vi "Main.vi"(8 "error in":errorcluster caption="entrée d'erreur") -> (0 "error out":errorcluster caption="sortie d'erreur")   [LabVIEW 2026]
uses:
  FGV/TypeDef_Array_ChannelCluster.ctl
  FGV/TypeDef_FGV.ctl
panel:
  in  "Arrêter":bool
  in  "Channel_Cluster_Array IN":T1 {"Filter" items=["447/60", "475/35", "525/50", "600/37", "647/57", "647LP"]; "Exposure time (s)" min=0.0 max=5.0 step=0.01; "Power (%)" max=100 step=1}
  out "Waveform Graph":waveform(dbl)[](graph)=[{"t0"=timestamp(0 s since 1904-01-01), "dt"=1e-05, "Y"=array[75000 elements]}, {"t0"=timestamp(0 s since 1904-01-01), "dt"=1e-05, "Y"=array[75000 elements]}, {"t0"=timestamp(0 s since 1904-01-01), "dt"=1e-05, "Y"=array[75000 elements]}, {"t0"=timestamp(0 s since 1904-01-01), "dt"=1e-05, "Y"=array[75000 elements]}]
  out "DO WF OUT":digitalwaveform(graph)
  out "Waveform Graph 2":waveform(dbl)[](graph)=[{"t0"=timestamp(0 s since 1904-01-01), "dt"=1e-05, "Y"=array[75000 elements]}, {"t0"=timestamp(0 s since 1904-01-01), "dt"=1e-05, "Y"=array[75000 elements]}, {"t0"=timestamp(0 s since 1904-01-01), "dt"=1e-05, "Y"=array[75000 elements]}]
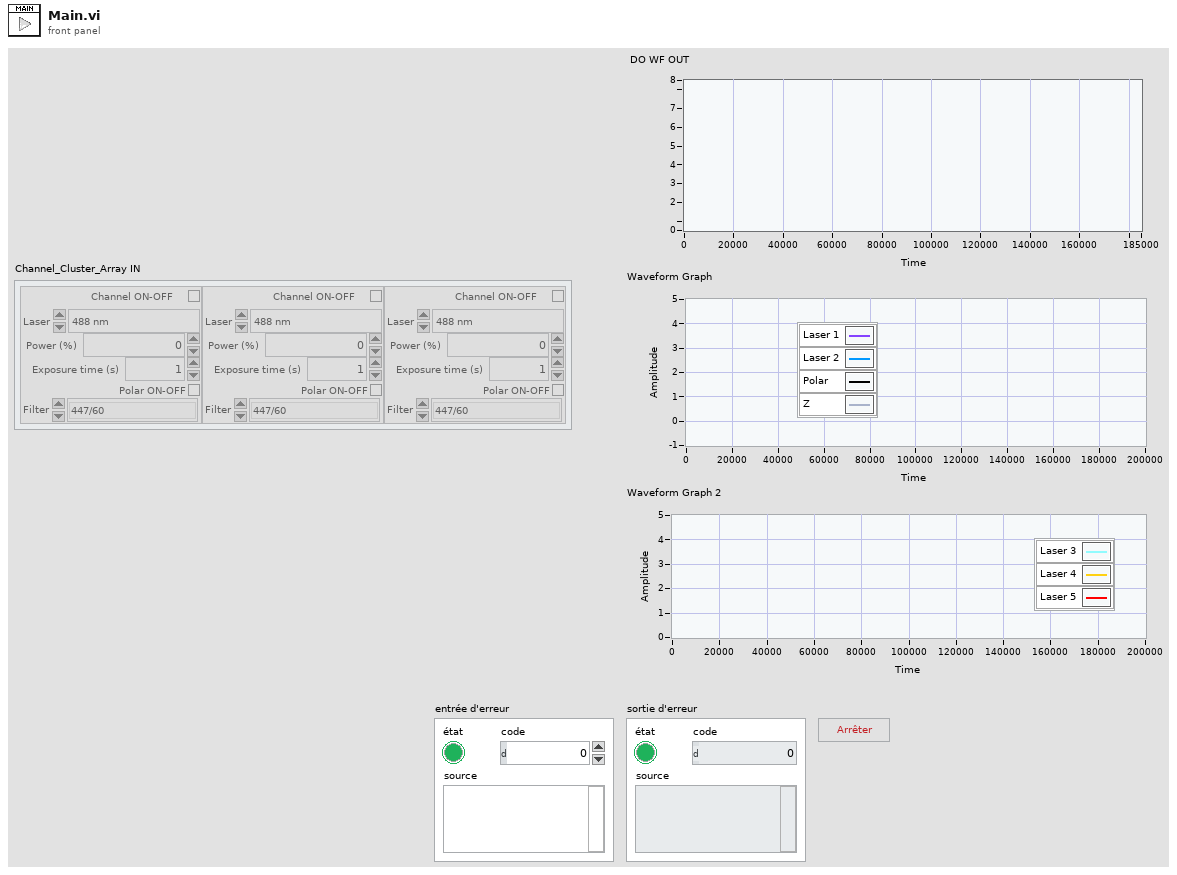
[diagram p1: front panel]
types:
  T1 = typedef "TypeDef_Array_ChannelCluster.ctl" = cluster{"Laser":enum16{"405 nm", "455 nm", "488 nm", "561 nm", "640 nm"}, "Power (%)":u8, "Exposure time (s)":dbl, "Channel ON-OFF":bool, "Polar ON-OFF":bool, "Filter":u16}[]
  T2 = typedef "TypeDef_FGV.ctl" = enum16{"Initialize", "Write", "Read", "Read_File", "Write_to_File"}
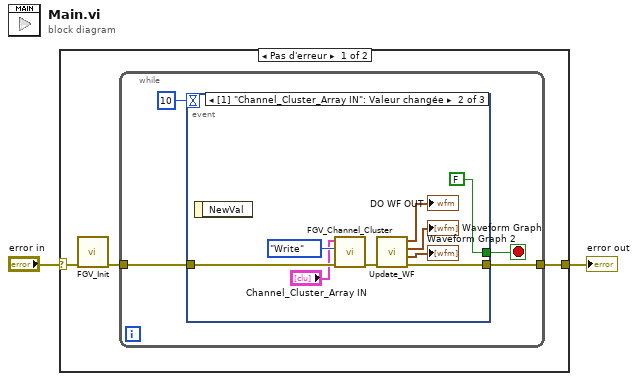
[diagram p0: block diagram]
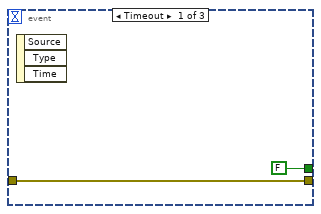
[diagram p2: hidden frame]
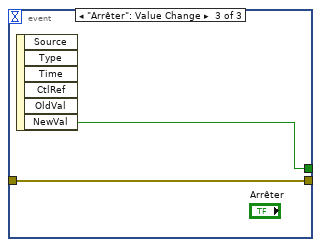
[diagram p3: hidden frame]
diagram:
  n1 = case shown="Pas d'erreur" "error in" {
    selector: "error in" -> [w3 w23]
    tunnel: [w5 w23] -> w1
    frame No Error {
      n2 = call "FGV_Init.vi"("error in"=w3) -> ("error out"=w4:errorcluster)  [unwired: 10 in]
      n3 = while {
        tunnel: [w7] -> w5
        tunnel: w4 -> [w6]
        stop <- w9 stop-if-true
        n4 = event shown="[1] \"Channel_Cluster_Array IN\": Valeur changée" {
          selector: _ -> [_ _ _]
          dyn-events: _ -> [_ _ _]
          timeout: 10 -> [_ _ _]
          tunnel: [FALSE ("NewVal") FALSE w22] -> w9
          tunnel: [w10 w13 w21] -> w7
          tunnel: w6 -> [w10 w14 w21]
          event Timeout {
            n5 = event-data() -> ()  [unwired: 1 in, 3 out]
          }
          event Value Change {
            n6 = event-data() -> ()  [unwired: 1 in, 1 out]
            n7 = call "FGV_Channel_Cluster.vi"("error in"=w14, "Action"=TypeDef_FGV."Write", "Channel_Cluster_Array IN"="Channel_Cluster_Array IN") -> ("error out"=w16:errorcluster)  [unwired: 7 in, 1 out]
            n8 = call "Update_WF.vi"("entrée d'erreur (pas d'erreur)"=w16) -> ("sortie d'erreur"=w13:errorcluster, "Waveform Graph 2"=→"Waveform Graph 2":waveform(dbl)[], "Waveform Graph"=→"Waveform Graph":waveform(dbl)[], "DO WF OUT"=→"DO WF OUT":digitalwaveform)  [unwired: 7 in]
          }
          event "Arrêter": Value Change {
            n9 = event-data() -> ("NewVal"=w22:bool)  [unwired: 1 in, 5 out]
          }
        }
      }
    }
    frame Error {
    }
  }
  "error out" <- w1
